vi "LiveMode.vi"() -> ()   [LabVIEW 2019]
uses:
  <userlib>/AndorSDK3/Data/GetPixelData16.vi
panel:
  in  "Apply Settings":bool
  in  "Centre AOI":bool
  in  "AOI Width":i64
  in  "AOI Height":i64
  out "Ready":bool
  in  "Run":bool
  in  "error":errorcluster
  out "Pixel Encoding":string
  out "Intensity Graph":u16[][](graph)
  out "AOIStride":i64
  in  "PreAmp Gain Control":string(combo)
  out "PixelData":u16[](array[numeric])
  out "ByteData":u8[](array[numeric])
  in  "ExposureTime":dbl=0.1
  out "ImageSizeBytes":i64
  out "Handle":i32
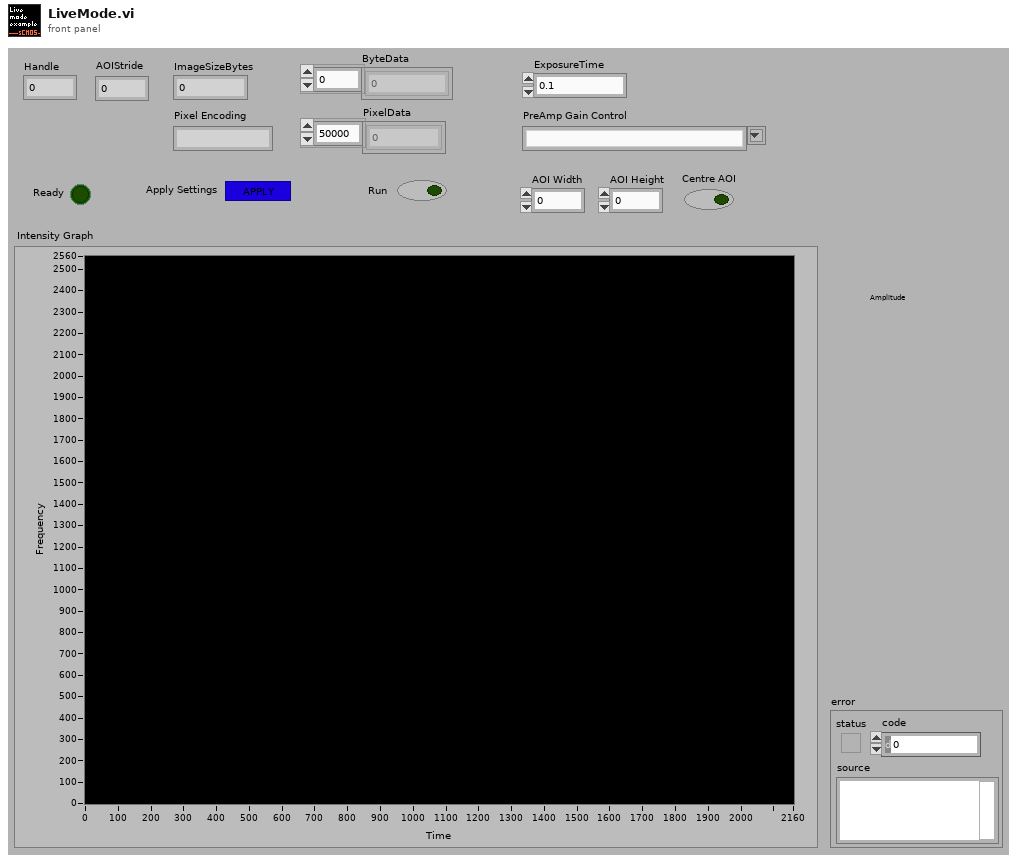
[diagram p1: front panel]
types:
  T1 = enum8{"Enabled", "Disabled", "Disabled and Grayed Out"}
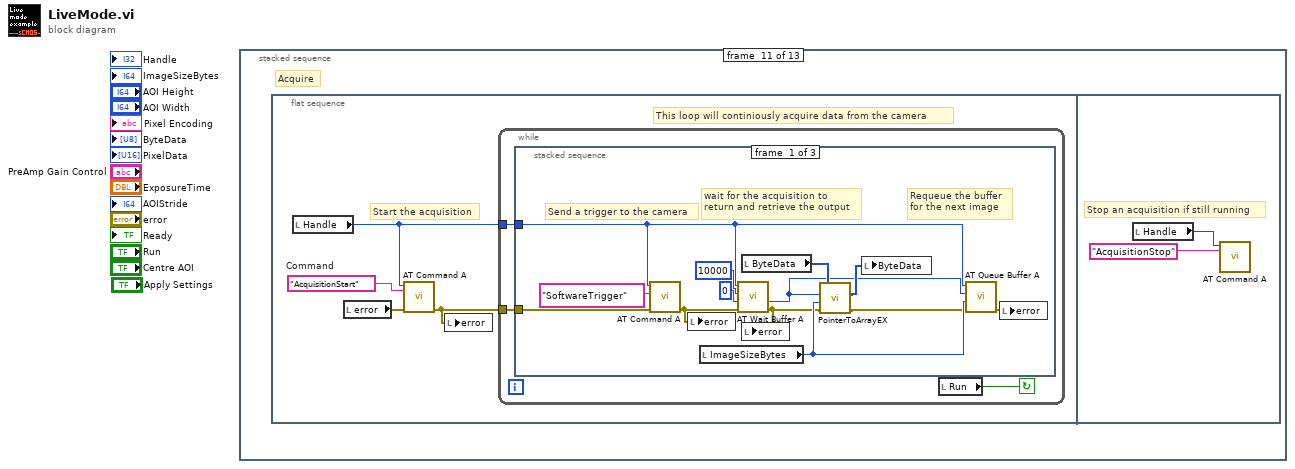
[diagram p0: block diagram]
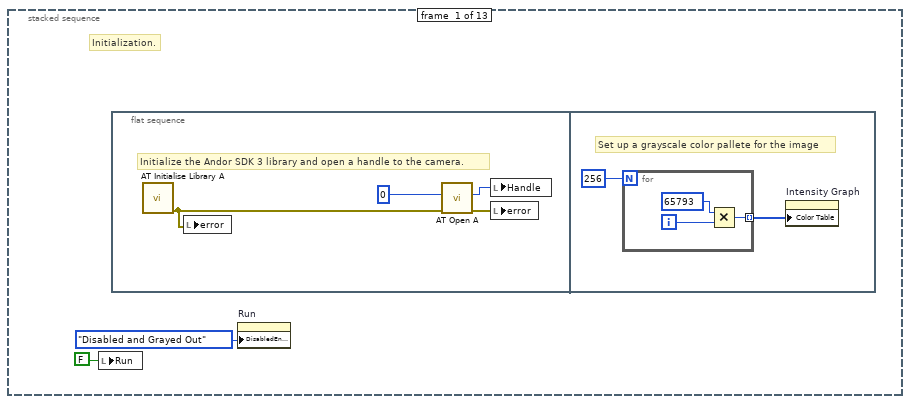
[diagram p2: hidden frame]
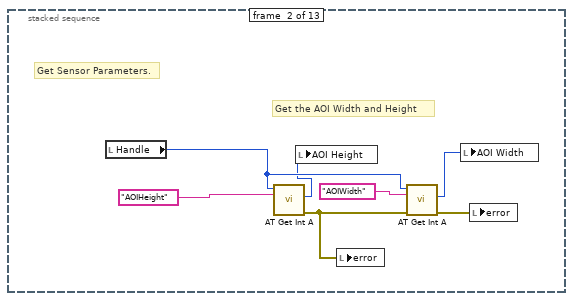
[diagram p3: hidden frame]
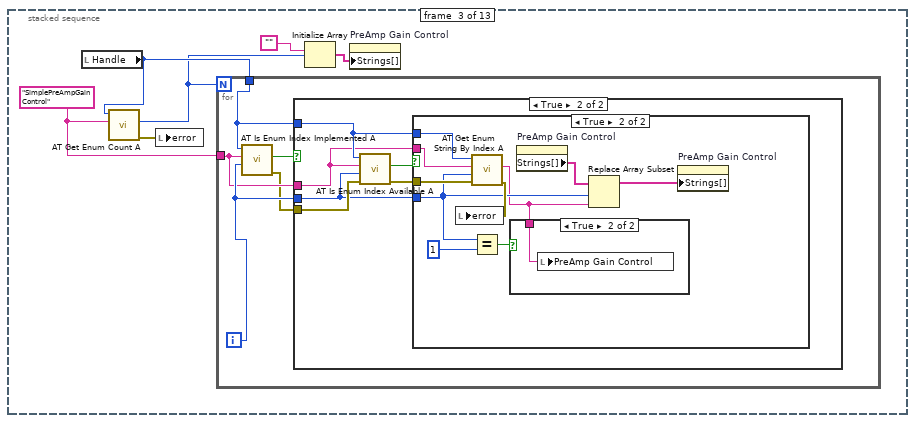
[diagram p4: hidden frame]
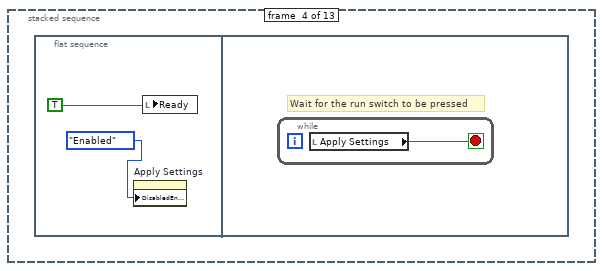
[diagram p8: hidden frame]
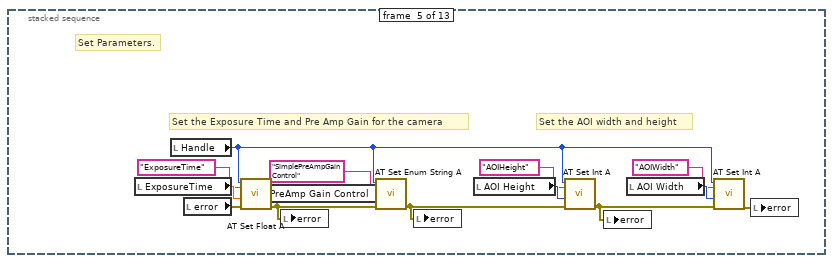
[diagram p9: hidden frame]
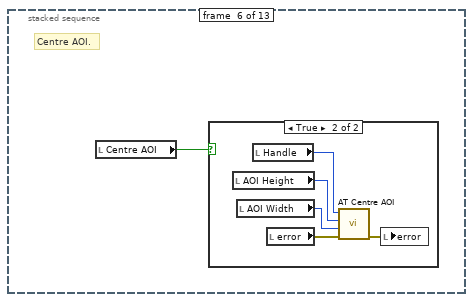
[diagram p10: hidden frame]
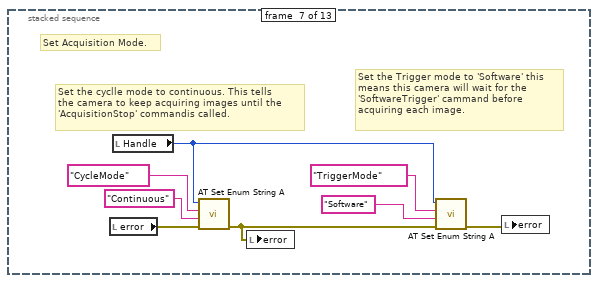
[diagram p12: hidden frame]
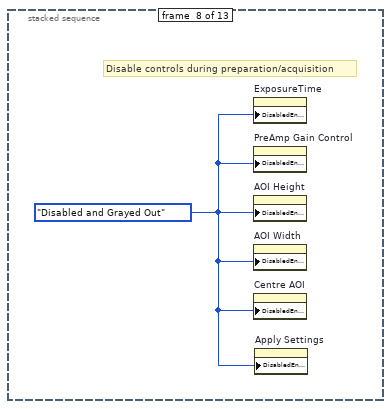
[diagram p13: hidden frame]
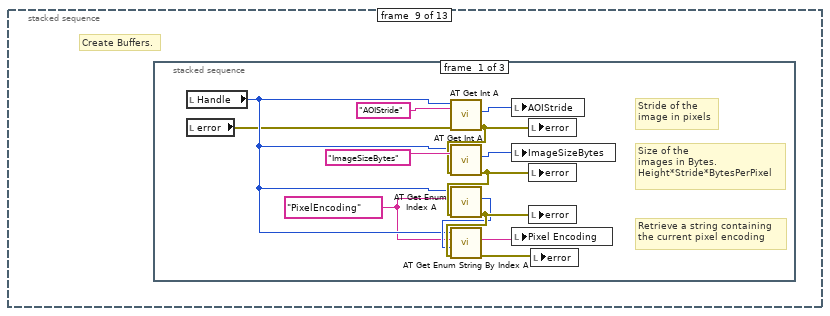
[diagram p14: hidden frame]
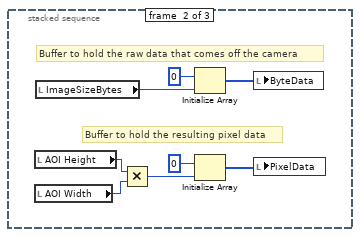
[diagram p15: hidden frame]
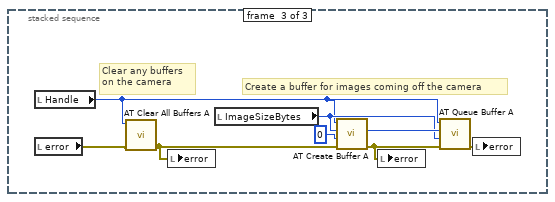
[diagram p16: hidden frame]
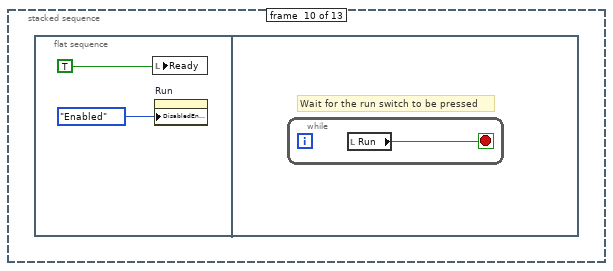
[diagram p17: hidden frame]
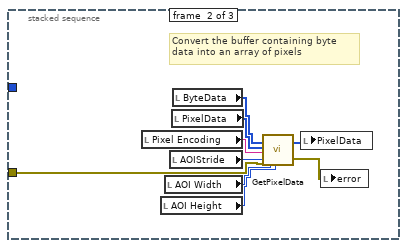
[diagram p18: hidden frame]
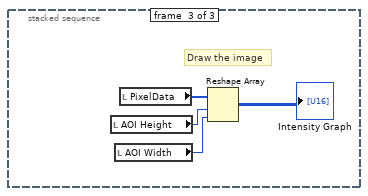
[diagram p19: hidden frame]
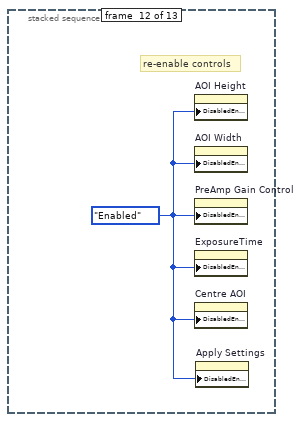
[diagram p20: hidden frame]
diagram:
  n1 = stacked-sequence {
    frame #0 {
      # "Initialization."
      n2 = local write "Run"(FALSE ("Run")) -> ()
      n3 = flat-sequence {
        frame #0 {
          # "Initialize the Andor SDK 3 library and open a handle to the camera."
          n4 = call <userlib>:"AT Initialise Library A.vi"() -> ("error out"=w4:errorcluster)  [unwired: 10 in, 1 out]
          n5 = local write "error"(w4) -> ()
          n6 = call <userlib>:"AT Open A.vi"("error in (no error)"=w4, "CameraIndex"=0) -> ("error out"=w3:errorcluster, "Handle"=w5:i32)  [unwired: 7 in, 1 out]
          n7 = local write "Handle"(w5) -> ()
          n8 = local write "error"(w3) -> ()
        }
        frame #1 {
          # "Set up a grayscale color pallete for the image"
          n9 = for {
            N: 256 -> [_]
            tunnel: [w10] -> w7 mode=indexing
            i -> [w11]
            n10 = Multiply(x=65793, y=w11) -> (x*y=w10:i32)
          }
          n11 = property on="Intensity Graph" class="IntGraph (strict)"("Color Table"=w7) -> ()  [unwired: 2 in, 2 out]
        }
      }
      n12 = property on="Run" class="Bool (strict)"("DisabledEnum"=T1."Disabled and Grayed Out" ("Disabled")) -> ()  [unwired: 2 in, 2 out]
    }
    frame #1 {
      # "Get the AOI Width and Height"
      # "Get Sensor Parameters."
      n13 = local read "Handle"() -> (w15:i32)
      n14 = call <userlib>:"AT Get Int A.vi"("Feature"="AOIHeight" ("Integer feature 2"), "Handle"=w15) -> ("error out"=w14:errorcluster, "Value"=w12:i64)  [unwired: 7 in, 1 out]
      n15 = local write "AOI Height"(w12) -> ()
      n16 = local write "error"(w14) -> ()
      n17 = call <userlib>:"AT Get Int A.vi"("error in (no error)"=w14, "Feature"="AOIWidth" ("Integer feature"), "Handle"=w15) -> ("error out"=w18:errorcluster, "Value"=w13:i64)  [unwired: 6 in, 1 out]
      n18 = local write "AOI Width"(w13) -> ()
      n19 = local write "error"(w18) -> ()
    }
    frame #2 {
      w19 = "SimplePreAmpGainControl" ("Enum feature")
      n20 = local read "Handle"() -> (w23:i32)
      n21 = call <userlib>:"AT Get Enum Count A.vi"("Feature"=w19, "Handle"=w23) -> ("error out"=w24:errorcluster, "Count"=w22:i32)  [unwired: 7 in, 1 out]
      n22 = local write "error"(w24) -> ()
      n23 = for {
        N: w22 -> [_]
        tunnel: w23 -> [w26]
        tunnel: w19 -> [w27]
        i -> [w28]
        n24 = call <userlib>:"AT Is Enum Index Implemented A.vi"("Index"=w28, "Feature"=w27, "Handle"=w26) -> ("error out"=w25:errorcluster, "Implemented"=w29:bool)  [unwired: 6 in, 1 out]
        n25 = case shown="True" w29 {
          tunnel: w28 -> [_ w31]
          tunnel: w27 -> [_ w32]
          tunnel: w26 -> [_ w33]
          tunnel: w25 -> [_ w35]
          frame False {
          }
          frame True {
            n26 = call <userlib>:"AT Is Enum Index Available A.vi"("error in (no error)"=w35, "Index"=w31, "Feature"=w32, "Handle"=w33) -> ("error out"=w30:errorcluster, "Available"=w34:bool)  [unwired: 5 in, 1 out]
            n27 = case shown="True" w34 {
              tunnel: w33 -> [_ w45]
              tunnel: w32 -> [_ w44]
              tunnel: w31 -> [_ w41]
              tunnel: w30 -> [_ w43]
              frame False {
              }
              frame True {
                n28 = call <userlib>:"AT Get Enum String By Index A.vi"("error in (no error)"=w43, "Index"=w41, "Feature"=w44, "Handle"=w45) -> ("error out"=w42:errorcluster, "String"=w38:string)  [unwired: 5 in, 1 out]
                n29 = local write "error"(w42) -> ()
                n30 = Equal?(x=w41, y=1) -> (x = y?=w39:bool)
                n31 = case shown="True" w39 {
                  tunnel: w38 -> [_ w46]
                  frame False {
                  }
                  frame True {
                    n32 = local write "PreAmp Gain Control"(w46) -> ()
                  }
                }
                n33 = property on="PreAmp Gain Control" class="CmbBox"() -> ("Strings[]"=w37:string[])  [unwired: 2 in, 2 out]
                n34 = Replace Array Subset(array=w37, new element=w38, index=w41) -> (w36:string[])
                n35 = property on="PreAmp Gain Control" class="CmbBox"("Strings[]"=w36) -> ()  [unwired: 2 in, 2 out]
              }
            }
          }
        }
      }
      n36 = Initialize Array("", w22) -> (w20:string[])
      n37 = property on="PreAmp Gain Control" class="CmbBox"("Strings[]"=w20) -> ()  [unwired: 2 in, 2 out]
    }
    frame #3 {
      n38 = flat-sequence {
        frame #0 {
          n39 = property on="Apply Settings" class="Bool (strict)"("DisabledEnum"=T1."Enabled" ("Disabled")) -> ()  [unwired: 2 in, 2 out]
          n40 = local write "Ready"(TRUE ("Ready")) -> ()
        }
        frame #1 {
          # "Wait for the run switch to be pressed"
          n41 = while {
            stop <- w49 stop-if-true
            n42 = local read "Apply Settings"() -> (w49:bool)
          }
        }
      }
    }
    frame #4 {
      # "Set the AOI width and height"
      # "Set the Exposure Time and Pre Amp Gain for the camera"
      # "Set Parameters."
      n43 = local read "ExposureTime"() -> (w63:dbl)
      n44 = local read "Handle"() -> (w51:i32)
      n45 = local read "error"() -> (w59:errorcluster)
      n46 = call <userlib>:"AT Set Float A.vi"("error in (no error)"=w59, "Value"=w63, "Feature"="ExposureTime" ("ExposureTime"), "Hndl"=w51) -> ("error out"=w61:errorcluster)  [unwired: 6 in, 1 out]
      n47 = local read "PreAmp Gain Control"() -> (w62:string)
      n48 = local write "error"(w61) -> ()
      n49 = call <userlib>:"AT Set Enum String A.vi"("error in (no error)"=w61, "String"=w62, "Feature"="SimplePreAmpGainControl" ("Enum feature"), "Handle"=w51) -> ("error out"=w58:errorcluster)  [unwired: 6 in, 1 out]
      n50 = local write "error"(w58) -> ()
      n51 = local read "AOI Height"() -> (w55:i64)
      n52 = call <userlib>:"AT Set Int A.vi"("error in (no error)"=w58, "Value"=w55, "Feature"="AOIHeight" ("Integer feature"), "Handle"=w51) -> ("error out"=w56:errorcluster)  [unwired: 6 in, 1 out]
      n53 = local write "error"(w56) -> ()
      n54 = local read "AOI Width"() -> (w54:i64)
      n55 = call <userlib>:"AT Set Int A.vi"("error in (no error)"=w56, "Value"=w54, "Feature"="AOIWidth" ("Integer feature 2"), "Handle"=w51) -> ("error out"=w57:errorcluster)  [unwired: 6 in, 1 out]
      n56 = local write "error"(w57) -> ()
    }
    frame #5 {
      # "Centre AOI."
      n57 = local read "Centre AOI"() -> (w64:bool)
      n58 = case shown="True" w64 {
        frame False {
        }
        frame True {
          n59 = local read "AOI Height"() -> (w66:i64)
          n60 = local read "AOI Width"() -> (w67:i64)
          n61 = local read "Handle"() -> (w65:i32)
          n62 = local read "error"() -> (w68:errorcluster)
          n63 = call <userlib>:"AT Centre AOI.vi"("error in (no error)"=w68, "AOI Width"=w67, "AOI Height"=w66, "Handle"=w65) -> ("error out"=w69:errorcluster)  [unwired: 7 in]
          n64 = local write "error"(w69) -> ()
        }
      }
    }
    frame #6 {
      # "Set the Trigger mode to 'Software' this \nmeans this camera will wait for the \n'SoftwareTrigger' cammand before \nacquiring each image."
      # "Set the cyclle mode to continuous. This tells \nthe camera to keep acquiring images until the \n'AcquisitionStop' commandis called."
      # "Set Acquisition Mode."
      n65 = local read "error"() -> (w76:errorcluster)
      n66 = local read "Handle"() -> (w74:i32)
      n67 = call <userlib>:"AT Set Enum String A.vi"("error in (no error)"=w76, "String"="Continuous", "Feature"="CycleMode" ("Enum feature"), "Handle"=w74) -> ("error out"=w75:errorcluster)  [unwired: 6 in, 1 out]
      n68 = local write "error"(w75) -> ()
      n69 = call <userlib>:"AT Set Enum String A.vi"("error in (no error)"=w75, "String"="Software", "Feature"="TriggerMode" ("Enum feature"), "Handle"=w74) -> ("error out"=w72:errorcluster)  [unwired: 6 in, 1 out]
      n70 = local write "error"(w72) -> ()
    }
    frame #7 {
      w78 = T1."Disabled and Grayed Out" ("Disabled")
      # "Disable controls during preparation/acquisition"
      n71 = property on="ExposureTime" class="DigNum (strict)"("DisabledEnum"=w78) -> ()  [unwired: 2 in, 2 out]
      n72 = property on="PreAmp Gain Control" class="CmbBox"("DisabledEnum"=w78) -> ()  [unwired: 2 in, 2 out]
      n73 = property on="AOI Height" class="DigNum (strict)"("DisabledEnum"=w78) -> ()  [unwired: 2 in, 2 out]
      n74 = property on="AOI Width" class="DigNum (strict)"("DisabledEnum"=w78) -> ()  [unwired: 2 in, 2 out]
      n75 = property on="Centre AOI" class="Bool (strict)"("DisabledEnum"=w78) -> ()  [unwired: 2 in, 2 out]
      n76 = property on="Apply Settings" class="Bool (strict)"("DisabledEnum"=w78) -> ()  [unwired: 2 in, 2 out]
    }
    frame #8 {
      # "Create Buffers."
      n77 = stacked-sequence {
        frame #0 {
          w79 = "PixelEncoding" ("Enum feature")
          # "Retrieve a string containing \nthe current pixel encoding"
          # "Stride of the\nimage in pixels"
          # "Size of the\nimages in Bytes.\nHeight*Stride*BytesPerPixel"
          n78 = local read "Handle"() -> (w81:i32)
          n79 = local read "error"() -> (w80:errorcluster)
          n80 = call <userlib>:"AT Get Int A.vi"("error in (no error)"=w80, "Feature"="AOIStride" ("Integer feature"), "Handle"=w81) -> ("error out"=w87:errorcluster, "Value"=w91:i64)  [unwired: 6 in, 1 out]
          n81 = call <userlib>:"AT Get Int A.vi"("error in (no error)"=w87, "Feature"="ImageSizeBytes" ("Integer feature"), "Handle"=w81) -> ("error out"=w86:errorcluster, "Value"=w90:i64)  [unwired: 6 in, 1 out]
          n82 = call <userlib>:"AT Get Enum Index A.vi"("error in (no error)"=w86, "Feature"=w79, "Handle"=w81) -> ("error out"=w85:errorcluster, "Value"=w84:i32)  [unwired: 6 in, 1 out]
          n83 = call <userlib>:"AT Get Enum String By Index A.vi"("error in (no error)"=w85, "Index"=w84, "Feature"=w79, "Handle"=w81) -> ("error out"=w82:errorcluster, "String"=w83:string)  [unwired: 5 in, 1 out]
          n84 = local write "AOIStride"(w91) -> ()
          n85 = local write "ImageSizeBytes"(w90) -> ()
          n86 = local write "Pixel Encoding"(w83) -> ()
          n87 = local write "error"(w87) -> ()
          n88 = local write "error"(w86) -> ()
          n89 = local write "error"(w85) -> ()
          n90 = local write "error"(w82) -> ()
        }
        frame #1 {
          # "Buffer to hold the resulting pixel data"
          # "Buffer to hold the raw data that comes off the camera"
          n91 = local read "AOI Height"() -> (w97:i64)
          n92 = local read "AOI Width"() -> (w98:i64)
          n93 = local read "ImageSizeBytes"() -> (w93:i64)
          n94 = Multiply(x=w97, y=w98) -> (x*y=w92:i64)
          n95 = Initialize Array(u8 0, w93) -> (w95:u8[])
          n96 = Initialize Array(i64 0, w92) -> (w96:i64[])
          n97 = local write "ByteData"(w95) -> ()
          n98 = local write "PixelData"(w96) -> ()
        }
        frame #2 {
          # "Clear any buffers \non the camera"
          # "Create a buffer for images coming off the camera"
          n99 = local read "Handle"() -> (w100:i32)
          n100 = local read "error"() -> (w102:errorcluster)
          n101 = call <userlib>:"AT Clear All Buffers A.vi"("error in (no error)"=w102, "Handle"=w100) -> ("error out"=w101:errorcluster)  [unwired: 8 in, 1 out]
          n102 = local write "error"(w101) -> ()
          n103 = local read "ImageSizeBytes"() -> (w104:i64)
          n104 = call <userlib>:"AT Create Buffer A.vi"("error in (no error)"=w101, "Buffer"=0 ("Size"), "Size"=w104, "Handle"=w100) -> ("error out"=w106:errorcluster, "Buffer out"=w107:u64)  [unwired: 5 in, 1 out]
          n105 = local write "error"(w106) -> ()
          n106 = call <userlib>:"AT Queue Buffer A.vi"("error in (no error)"=w106, "PtrSize"=w104, "Ptr"=w107, "Handle"=w100) -> ("error out"=w103:errorcluster)  [unwired: 6 in, 1 out]
          n107 = local write "error"(w103) -> ()
        }
      }
    }
    frame #9 {
      n108 = flat-sequence {
        frame #0 {
          n109 = local write "Ready"(TRUE ("Ready")) -> ()
          n110 = property on="Run" class="Bool (strict)"("DisabledEnum"=T1."Enabled" ("Disabled")) -> ()  [unwired: 2 in, 2 out]
        }
        frame #1 {
          # "Wait for the run switch to be pressed"
          n111 = while {
            stop <- w110 stop-if-true
            n112 = local read "Run"() -> (w110:bool)
          }
        }
      }
    }
    frame #10 {
      # "Acquire"
      n113 = flat-sequence {
        frame #0 {
          w112 = "AcquisitionStart"  # Command
          # "This loop will continiously acquire data from the camera"
          # "Start the acquisition"
          n114 = local read "Handle"() -> (w114:i32)
          n115 = local read "error"() -> (w113:errorcluster)
          n116 = call <userlib>:"AT Command A.vi"("error in (no error)"=w113, "Feature"=w112, "Handle"=w114) -> ("error out"=w111:errorcluster)  [unwired: 7 in, 1 out]
          n117 = local write "error"(w111) -> ()
          n118 = while {
            tunnel: w114 -> [w116]
            tunnel: w111 -> [w117]
            stop <- w115 continue-if-true
            n119 = stacked-sequence {
              tunnel: w117 -> [w125 w131 _]
              tunnel: w116 -> [w126 _ _]
              frame #0 {
                # "Requeue the buffer\nfor the next image"
                # "Send a trigger to the camera"
                # "wait for the acquisition to \nreturn and retrieve the output"
                n120 = call <userlib>:"AT Command A.vi"("error in (no error)"=w125, "Feature"="SoftwareTrigger" ("Command"), "Handle"=w126) -> ("error out"=w124:errorcluster)  [unwired: 7 in, 1 out]
                n121 = local write "error"(w124) -> ()
                n122 = local read "ImageSizeBytes"() -> (w122:i64)
                n123 = call <userlib>:"AT Wait Buffer A.vi"("error in (no error)"=w124, "Input buffer"=u32 0, "Timeout"=u32 10000, "Handle"=w126) -> ("error out"=w119:errorcluster, "Output buffer"=w118:u64)  [unwired: 4 in, 2 out]
                n124 = local read "ByteData"() -> (w123:u8[])
                n125 = local write "error"(w119) -> ()
                n126 = call <userlib>:"PointerToArrayEX.vi"("Array in"=w123, "Pointer In"=w118, "Pointer Size"=w122, "error in (no error)"=w119) -> ("Array out"=w121:u8[], "error out"=w120:errorcluster)  [unwired: 4 in]
                n127 = local write "ByteData"(w121) -> ()
                n128 = call <userlib>:"AT Queue Buffer A.vi"("error in (no error)"=w120, "PtrSize"=w122, "Ptr"=w118, "Handle"=w126) -> ("error out"=w128:errorcluster)  [unwired: 6 in, 1 out]
                n129 = local write "error"(w128) -> ()
              }
              frame #1 {
                # "Convert the buffer containing byte \ndata into an array of pixels"
                n130 = local read "Pixel Encoding"() -> (w137:string)
                n131 = local read "AOI Height"() -> (w134:i64)
                n132 = local read "AOI Width"() -> (w135:i64)
                n133 = local read "AOIStride"() -> (w138:i64)
                n134 = local read "PixelData"() -> (w136:u16[])
                n135 = local read "ByteData"() -> (w132:u8[])
                n136 = call-poly <userlib>:"GetPixelData.vi"("Input buffer"=w132, "Output buffer in"=w136, "Pixel Encoding"=w137, "Stride"=w138, "error in (no error)"=w131, "Width"=w135, "Height"=w134) -> ("Output buffer out"=w139:u16[], "error out"=w133:errorcluster)  [unwired: 10 in, 1 out]
                n137 = local write "PixelData"(w139) -> ()
                n138 = local write "error"(w133) -> ()
              }
              frame #2 {
                # "Draw the image"
                n139 = local read "AOI Height"() -> (w142:i64)
                n140 = local read "AOI Width"() -> (w141:i64)
                n141 = local read "PixelData"() -> (w143:u16[])
                n142 = Reshape Array(w143, w142, w141) -> (→"Intensity Graph":u16[][])
              }
            }
            n143 = local read "Run"() -> (w115:bool)
          }
        }
        frame #1 {
          # "Stop an acquisition if still running"
          n144 = local read "Handle"() -> (w145:i32)
          n145 = call <userlib>:"AT Command A.vi"("Feature"="AcquisitionStop" ("Command"), "Handle"=w145) -> ()  [unwired: 8 in, 2 out]
        }
      }
    }
    frame #11 {
      w146 = T1."Enabled" ("Disabled")
      # "re-enable controls"
      n146 = property on="AOI Height" class="DigNum (strict)"("DisabledEnum"=w146) -> ()  [unwired: 2 in, 2 out]
      n147 = property on="AOI Width" class="DigNum (strict)"("DisabledEnum"=w146) -> ()  [unwired: 2 in, 2 out]
      n148 = property on="PreAmp Gain Control" class="CmbBox"("DisabledEnum"=w146) -> ()  [unwired: 2 in, 2 out]
      n149 = property on="ExposureTime" class="DigNum (strict)"("DisabledEnum"=w146) -> ()  [unwired: 2 in, 2 out]
      n150 = property on="Centre AOI" class="Bool (strict)"("DisabledEnum"=w146) -> ()  [unwired: 2 in, 2 out]
      n151 = property on="Apply Settings" class="Bool (strict)"("DisabledEnum"=w146) -> ()  [unwired: 2 in, 2 out]
    }
    frame #12 {
      # "Close the current camera handle and unload the library"
      # "ShutDown."
      n152 = local write "Apply Settings"(FALSE ("Apply Settings")) -> ()
      n153 = local write "Ready"(FALSE ("Ready")) -> ()
      n154 = local read "Handle"() -> (w149:i32)
      n155 = local read "error"() -> (w151:errorcluster)
      n156 = call <userlib>:"AT Flush A.vi"("error in (no error)"=w151, "Handle"=w149) -> ("error out"=w152:errorcluster)  [unwired: 8 in, 1 out]
      n157 = local write "error"(w152) -> ()
      n158 = call <userlib>:"AT Close A.vi"("error in (no error)"=w152, "Handle"=w149) -> ("error out"=w153:errorcluster)  [unwired: 8 in, 1 out]
      n159 = local write "error"(w153) -> ()
      n160 = call <userlib>:"AT Finalise Library A.vi"("error in (no error)"=w153) -> ("error out"=w150:errorcluster)  [unwired: 9 in, 1 out]
      n161 = local write "error"(w150) -> ()
    }
  }
